vi "RemoveBus.vi"(7 "BusNumber":i32, 8 "ErrorIn":errorcluster[](array[cluster]), 11 "Bus.lvclass":refnum<class "Bus.lvclass">) -> (0 "ErrorOut":errorcluster[](array[cluster]), 3 "Bus.lvclass":refnum<class "Bus.lvclass">)   [LabVIEW 2018, in "Bus.lvclass"]
uses:
  Bus.lvclass
  Bus.lvclass/Bus.ctl
  TestClass/Test.lvclass/Test.ctl
  Accessors/Write Test.vi
  Accessors/Write BusNumber.vi
  TestClass/Accessors/Read ErrorSeverity.vi
  Accessors/Read Test.vi
  Accessors/Read BusNumber.vi
  <vilib>/Utility/error.llb/Error Cluster From Error Code.vi
  TestClass/Test.lvclass
  <vilib>/ErrorRing/Error Ring.xnode
  <userlib>/NIST/NISTErrorLib/NISTErrorLib.lvlib
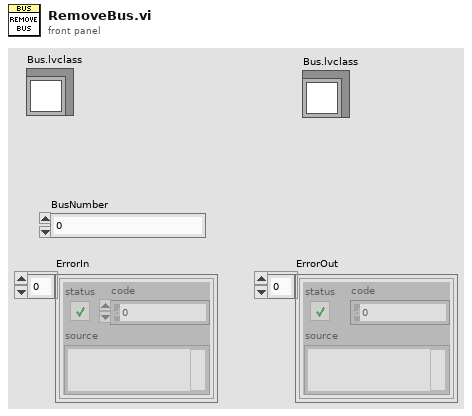
[diagram p1: front panel]
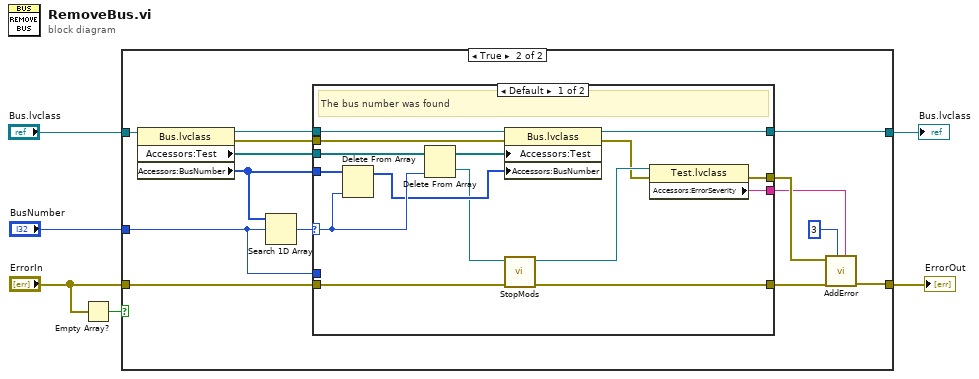
[diagram p0: block diagram]
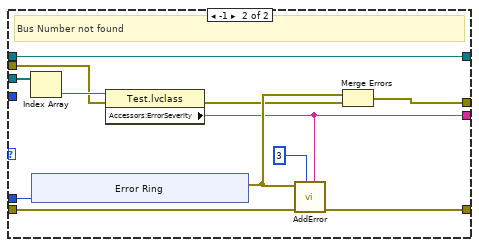
[diagram p3: hidden frame]
diagram:
  n1 = Empty Array?(array="ErrorIn") -> (empty?=w6:bool)
  n2 = case shown="True" w6 {
    tunnel: "ErrorIn" -> [w8 w18]
    tunnel: [w8 w11] -> w4
    tunnel: "Bus.lvclass" -> [w7 w22]
    tunnel: [w7 w15] -> w2
    tunnel: "BusNumber" -> [_ w20]
    frame False {
    }
    frame True {
      n3 = property class="Bus.lvclass"(reference=w22) -> (reference out=w17:refnum<class "Bus.lvclass">, error out=w14:errorcluster, "Accessors:Test"=w19:refnum<class "Test.lvclass">[], "Accessors:BusNumber"=w16:i32[])  [unwired: 1 in]
      n4 = Search 1D Array(1D array=w16, element=w20) -> (index of element=w21:i32)  [unwired: 1 in]
      n5 = case shown="Default" w21 {
        selector: w21 -> [w35 _]
        tunnel: w20 -> [_ w49]
        tunnel: w19 -> [w36 w48]
        tunnel: w18 -> [w29 w46]
        tunnel: [w28 w44] -> w12
        tunnel: w17 -> [w34 w43]
        tunnel: w16 -> [w37 _]
        tunnel: [w33 w43] -> w15
        tunnel: w14 -> [w27 w42]
        tunnel: [w23 w39] -> w10
        tunnel: [w25 w40] -> w9
        frame Default {
          # "The bus number was found"
          n6 = Delete From Array(array=w37, index=w35) -> (array with subset deleted=w32:i32[])  [unwired: 1 in, 1 out]
          n7 = Delete From Array(array=w36, index=w35) -> (deleted portion=w30:refnum<class "Test.lvclass">, array with subset deleted=w31:refnum<class "Test.lvclass">[])  [unwired: 1 in]
          n8 = property class="Bus.lvclass"(reference=w34, error in=w27, "Accessors:Test"=w31, "Accessors:BusNumber"=w32) -> (reference out=w33:refnum<class "Bus.lvclass">, error out=w24:errorcluster)
          n9 = call "StopMods.vi"("ErrorArray"=w29, "Test.lvclass"=w30) -> ("ErrorArray"=w28:errorcluster[], "Test.lvclass"=w26:refnum<class "Test.lvclass">)  [unwired: 8 in]
          n10 = property class="Test.lvclass"(reference=w26, error in=w24) -> (error out=w23:errorcluster, "Accessors:ErrorSeverity"=w25:string)  [unwired: 1 out]
        }
        frame -1 {
          # "Bus Number not found"
          n11 = Index Array(array=w48) -> (element=w47:refnum<class "Test.lvclass">)  [unwired: 1 in]
          n12 = xnode "Error Ring"("parameter 0"=w49) -> ("error out"=w41:errorcluster)
          n13 = property class="Test.lvclass"(reference=w47, error in=w42) -> (error out=w38:errorcluster, "Accessors:ErrorSeverity"=w40:string)  [unwired: 1 out]
          n14 = call <userlib>:"AddError.vi"("Severity"=w40, "Priority"=u8 3, "ErrorArray"=w46, "error in (no error)"=w41) -> ("ErrorArray"=w44:errorcluster[])  [unwired: 6 in, 1 out]
          n15 = Merge Errors(w41, w38) -> (w39:errorcluster)
        }
      }
      n16 = call <userlib>:"AddError.vi"("Severity"=w9, "Priority"=u8 3, "ErrorArray"=w12, "error in (no error)"=w10) -> ("ErrorArray"=w11:errorcluster[])  [unwired: 6 in, 1 out]
    }
  }
  "Bus.lvclass" <- w2
  "ErrorOut" <- w4
